vi "公式复合写入.vi"(11 "公式":cluster{"X^2":dbl, "X":dbl, "b":dbl}) -> ()   [LabVIEW 2016, in "斯坦道氨氮.lvlib"]
uses:
  <vilib>/Utility/miscctls.llb/LVPointTypeDef.ctl
panel:
  out "连接的字符串":string
  in  "参数下拉列表":enum16{"COD", "氨氮", "总氮", "总磷"}(ring)
  in  "量程下拉列表":enum16{"低量程", "高量程"}(ring)
  in  "取消":bool
  in  "确认":bool
  in  "加标回收":bool
  in  "标样核查":bool
  in  "跨度核查":bool
  in  "空白核查":bool
  in  "水样测量":bool=TRUE
  # "请选择要写入的参数"
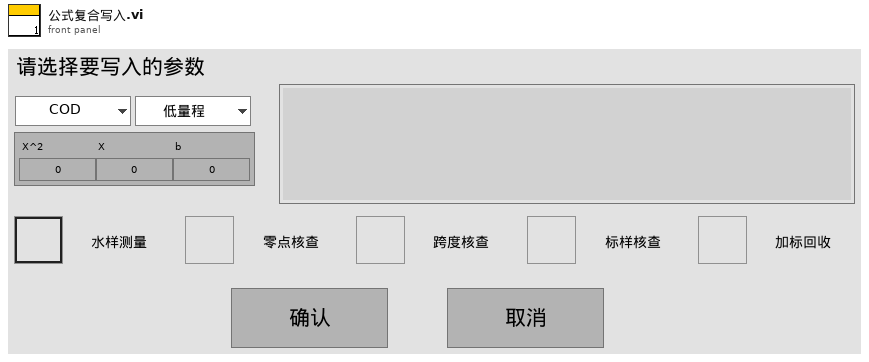
[diagram p1: front panel]
types:
  T1 = typedef "LVPointTypeDef.ctl" = cluster{"Horizontal":i16, "Vertical":i16}
  T2 = cluster{"COD":bool, "氨氮":bool, "总氮":bool, "总磷":bool}
  T3 = cluster{"测量量程":dbl, "测量精度":dbl, "测量间隔":dbl, "消解温度":dbl, "消解时长":dbl, "空白校准时间":timestamp, "曲线截距":dbl, "曲线斜率":dbl, "测量检出限":dbl, "测量信号值":dbl, "线性相关系数":dbl, "二次多项式系数":dbl, "标样校准时间":timestamp, "稀释倍数":dbl, "三项式系数":dbl, "空白标定系数":dbl, "量程系数":dbl, "F0/ORPA":dbl, "F1/ORPB":dbl, "F2/ORPK":dbl, "F3":dbl, "F4":dbl, "F5":dbl, "F6":dbl, "F7":dbl, "X0/滴定数":dbl, "量程":dbl}
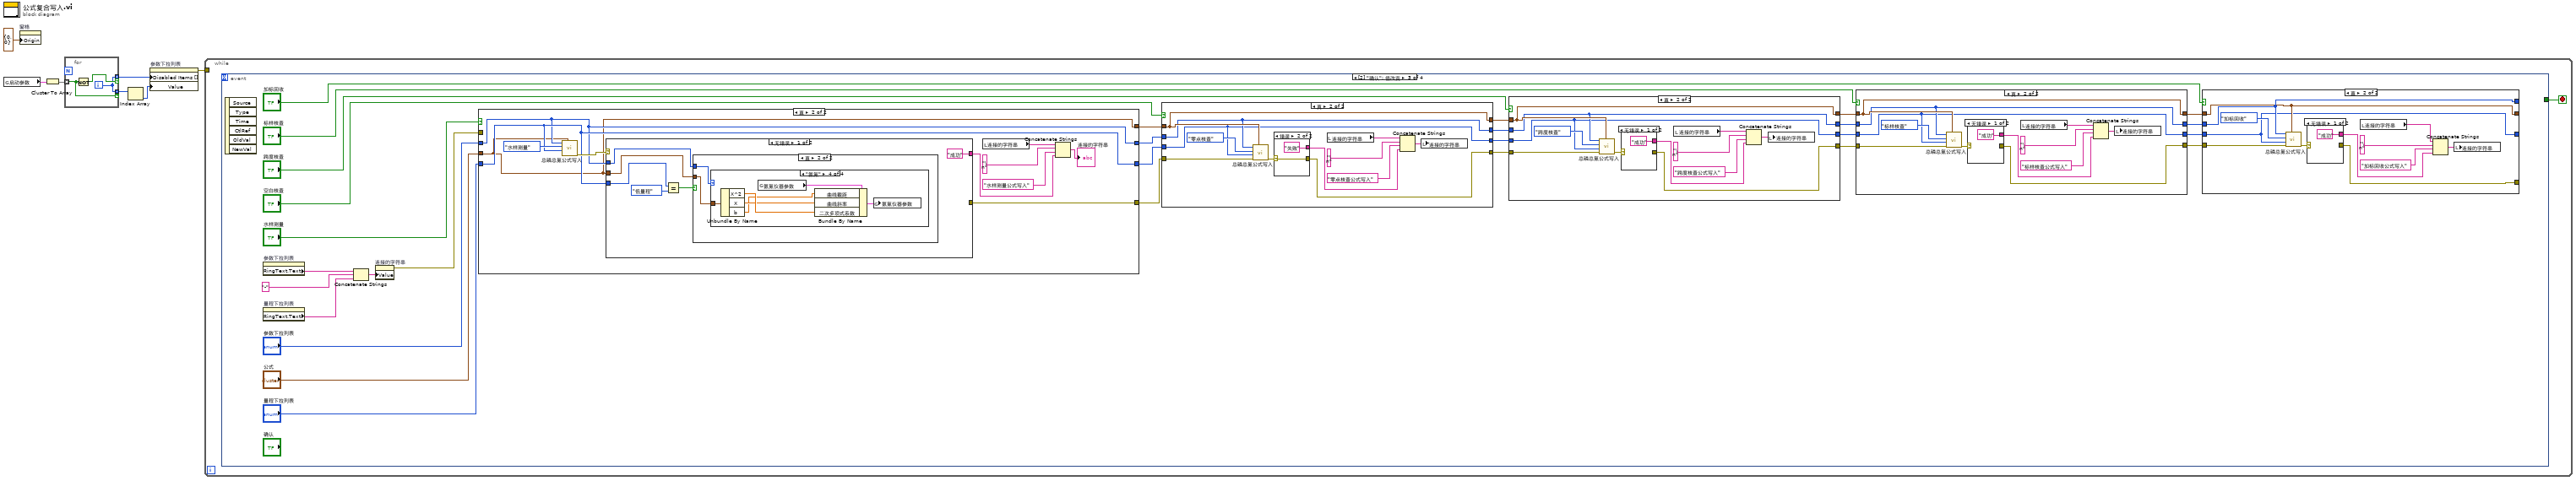
[diagram p0: block diagram]
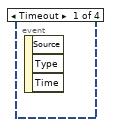
[diagram p2: hidden frame]
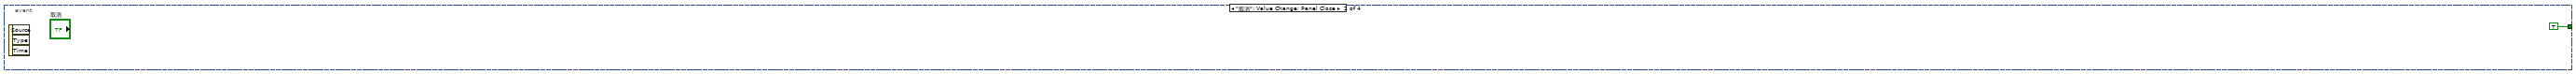
[diagram p3: hidden frame]
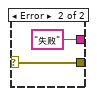
[diagram p5: hidden frame]
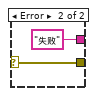
[diagram p7: hidden frame]
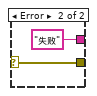
[diagram p9: hidden frame]
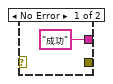
[diagram p11: hidden frame]
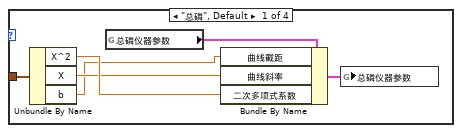
[diagram p14: hidden frame]
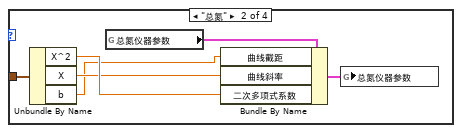
[diagram p15: hidden frame]
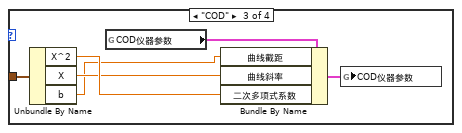
[diagram p16: hidden frame]
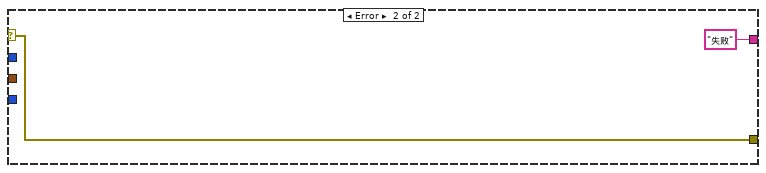
[diagram p17: hidden frame]
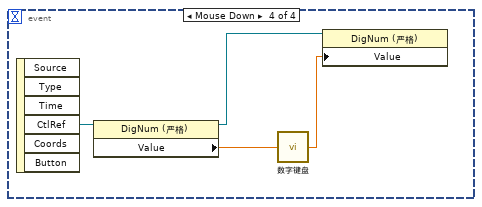
[diagram p18: hidden frame]
diagram:
  n1 = global read "总磷总氮断电保存全局变量.vi" "启动参数"() -> (w6:T2)
  n2 = property on="窗格" class="Pane"("Origin"=T1 {"Horizontal"=0, "Vertical"=0} ("原点")) -> ()  [unwired: 2 in, 2 out]
  n3 = Cluster To Array(cluster=w6) -> (array=w5:bool[])
  n4 = for {
    tunnel: w5 -> [w8] mode=indexing
    tunnel: [w9] -> w4 mode=indexing if=w10
    tunnel: [w9] -> w3 mode=indexing if=w8
    i -> [w9]
    n5 = Not(x=w8) -> (.not. x?=w10:bool)
  }
  n6 = Index Array(array=w3) -> (element=w2:i32)  [unwired: 1 in]
  n7 = property on="参数下拉列表" class="Enum (严格)"("Disabled Items []"=w4, "Value"=w2) -> (error out=w1:errorcluster)  [unwired: 2 in, 1 out]
  n8 = while {
    tunnel: w1 -> [_]
    stop <- w11 stop-if-true
    n9 = event shown="[2] \"确认\": 值改变" {
      selector: _ -> [_ _ _ _]
      dyn-events: _ -> [_ _ _ _]
      timeout: _ -> [_ _ _ _]
      tunnel: [_ TRUE _ _] -> w11
      event Timeout {
        n10 = event-data() -> ()  [unwired: 1 in, 3 out]
      }
      event "取消": Value Change; Panel Close {
        n11 = event-data() -> ()  [unwired: 1 in, 3 out]
      }
      event "确认": Value Change {
        n12 = event-data() -> ()  [unwired: 1 in, 6 out]
        n13 = property on="参数下拉列表" class="Enum (严格)"() -> ("RingText.Text"=w15:string)  [unwired: 2 in, 2 out]
        n14 = property on="量程下拉列表" class="Enum (严格)"() -> ("RingText.Text"=w14:string)  [unwired: 2 in, 2 out]
        n15 = Concatenate Strings(w15, "-" ("字符串"), w14) -> (w16:string)
        n16 = property on="连接的字符串" class="Str"("Value"=w16) -> (error out=w17:errorcluster)  [unwired: 2 in, 1 out]
        n17 = case shown="真" "水样测量" {
          tunnel: "公式" -> [w116 w117]
          tunnel: "参数下拉列表" -> [w115 w118]
          tunnel: "量程下拉列表" -> [w114 w119]
          tunnel: [w116 w117] -> w37
          tunnel: [w115 w118] -> w36
          tunnel: [w114 w119] -> w35
          tunnel: [_ w125] -> w19
          tunnel: w17 -> [_ _]
          frame False {
          }
          frame True {
            n18 = call "总磷总氮公式写入.vi"("公式"=w117, "量程"=w119, "测量模式"=enum16{"水样测量", "零点核查", "跨度核查", "标样核查", "加标回收"}."水样测量", "测量参数"=w118) -> ("error out"=w126:errorcluster)  [unwired: 7 in]
            n19 = case shown="无错误" w126 {
              selector: w126 -> [_ w161]
              tunnel: [_ w161] -> w125
              tunnel: ["成功" "失败"] -> w124
              tunnel: w119 -> [w132 _]
              tunnel: w118 -> [w129 _]
              tunnel: w117 -> [w128 _]
              frame No Error {
                n20 = Equal?(x=w132, y=enum16{"低量程", "高量程"}."低量程") -> (x = y?=w130:bool)
                n21 = case shown="真" w130 {
                  tunnel: w129 -> [_ w135]
                  tunnel: w128 -> [_ w134]
                  frame False {
                  }
                  frame True {
                    n22 = case shown="\"氨氮\"" w135 {
                      tunnel: w134 -> [w136 w142 w148 w154]
                      frame "总磷", Default {
                        n23 = Unbundle By Name(w136) -> ("X^2"=w139:dbl, "X"=w138:dbl, "b"=w137:dbl)
                        n24 = global read "总磷总氮断电保存全局变量.vi" "总磷仪器参数"() -> (w140:T3)
                        n25 = Bundle By Name(cluster=w140, "曲线截距"=w137, "曲线斜率"=w138, "二次多项式系数"=w139) -> (w141:T3)
                        n26 = global write "总磷总氮断电保存全局变量.vi" "总磷仪器参数"(w141) -> ()
                      }
                      frame "总氮" {
                        n27 = Unbundle By Name(w142) -> ("X^2"=w145:dbl, "X"=w144:dbl, "b"=w143:dbl)
                        n28 = global read "总磷总氮断电保存全局变量.vi" "总氮仪器参数"() -> (w146:T3)
                        n29 = Bundle By Name(cluster=w146, "曲线截距"=w143, "曲线斜率"=w144, "二次多项式系数"=w145) -> (w147:T3)
                        n30 = global write "总磷总氮断电保存全局变量.vi" "总氮仪器参数"(w147) -> ()
                      }
                      frame "COD" {
                        n31 = Unbundle By Name(w148) -> ("X^2"=w151:dbl, "X"=w150:dbl, "b"=w149:dbl)
                        n32 = global read "总磷总氮断电保存全局变量.vi" "COD仪器参数"() -> (w152:T3)
                        n33 = Bundle By Name(cluster=w152, "曲线截距"=w149, "曲线斜率"=w150, "二次多项式系数"=w151) -> (w153:T3)
                        n34 = global write "总磷总氮断电保存全局变量.vi" "COD仪器参数"(w153) -> ()
                      }
                      frame "氨氮" {
                        n35 = Unbundle By Name(w154) -> ("X^2"=w157:dbl, "X"=w156:dbl, "b"=w155:dbl)
                        n36 = global read "总磷总氮断电保存全局变量.vi" "氨氮仪器参数"() -> (w158:T3)
                        n37 = Bundle By Name(cluster=w158, "曲线截距"=w155, "曲线斜率"=w156, "二次多项式系数"=w157) -> (w159:T3)
                        n38 = global write "总磷总氮断电保存全局变量.vi" "氨氮仪器参数"(w159) -> ()
                      }
                    }
                  }
                }
              }
              frame Error {
              }
            }
            n39 = local read "连接的字符串"() -> (w121:string)
            n40 = Concatenate Strings(w121, "\n" ("字符串"), "水样测量公式写入", w124) -> (→"连接的字符串":string)
          }
        }
        n41 = case shown="真" "空白核查" {
          tunnel: w37 -> [w98 w109]
          tunnel: w36 -> [w97 w108]
          tunnel: w35 -> [w96 w107]
          tunnel: [_ w102] -> w34
          tunnel: [w98 w109] -> w33
          tunnel: [w97 w108] -> w32
          tunnel: [w96 w107] -> w31
          tunnel: w19 -> [_ w106]
          frame False {
          }
          frame True {
            n42 = call "总磷总氮公式写入.vi"("公式"=w109, "error in (no error)"=w106, "量程"=w107, "测量模式"=enum16{"水样测量", "零点核查", "跨度核查", "标样核查", "加标回收"}."零点核查", "测量参数"=w108) -> ("error out"=w103:errorcluster)  [unwired: 6 in]
            n43 = case shown="错误" w103 {
              selector: w103 -> [_ w113]
              tunnel: [_ w113] -> w102
              tunnel: ["成功" "失败"] -> w104
              frame No Error {
              }
              frame Error {
              }
            }
            n44 = local read "连接的字符串"() -> (w101:string)
            n45 = Concatenate Strings(w101, "\n" ("字符串"), "零点核查公式写入", w104) -> (w99:string)
            n46 = local write "连接的字符串"(w99) -> ()
          }
        }
        n47 = case shown="真" "跨度核查" {
          tunnel: w33 -> [w80 w91]
          tunnel: w32 -> [w79 w90]
          tunnel: w31 -> [w78 w89]
          tunnel: [w80 w91] -> w30
          tunnel: [w79 w90] -> w28
          tunnel: [w78 w89] -> w27
          tunnel: w34 -> [_ w88]
          tunnel: [_ w81] -> w18
          frame False {
          }
          frame True {
            n48 = call "总磷总氮公式写入.vi"("公式"=w91, "error in (no error)"=w88, "量程"=w89, "测量模式"=enum16{"水样测量", "零点核查", "跨度核查", "标样核查", "加标回收"}."跨度核查", "测量参数"=w90) -> ("error out"=w82:errorcluster)  [unwired: 6 in]
            n49 = case shown="无错误" w82 {
              selector: w82 -> [_ w95]
              tunnel: [_ w95] -> w81
              tunnel: ["成功" "失败"] -> w83
              frame No Error {
              }
              frame Error {
              }
            }
            n50 = local read "连接的字符串"() -> (w85:string)
            n51 = Concatenate Strings(w85, "\n" ("字符串"), "跨度核查公式写入", w83) -> (w87:string)
            n52 = local write "连接的字符串"(w87) -> ()
          }
        }
        n53 = case shown="真" "标样核查" {
          tunnel: w30 -> [w62 w73]
          tunnel: w28 -> [w61 w72]
          tunnel: w27 -> [w60 w71]
          tunnel: [_ w63] -> w24
          tunnel: [w62 w73] -> w29
          tunnel: [w61 w72] -> w26
          tunnel: [w60 w71] -> w25
          tunnel: w18 -> [_ w70]
          frame False {
          }
          frame True {
            n54 = call "总磷总氮公式写入.vi"("公式"=w73, "error in (no error)"=w70, "量程"=w71, "测量模式"=enum16{"水样测量", "零点核查", "跨度核查", "标样核查", "加标回收"}."标样核查", "测量参数"=w72) -> ("error out"=w64:errorcluster)  [unwired: 6 in]
            n55 = case shown="无错误" w64 {
              selector: w64 -> [_ w77]
              tunnel: [_ w77] -> w63
              tunnel: ["成功" "失败"] -> w65
              frame No Error {
              }
              frame Error {
              }
            }
            n56 = local read "连接的字符串"() -> (w67:string)
            n57 = Concatenate Strings(w67, "\n" ("字符串"), "标样核查公式写入", w65) -> (w69:string)
            n58 = local write "连接的字符串"(w69) -> ()
          }
        }
        n59 = case shown="真" "加标回收" {
          tunnel: w29 -> [w44 w55]
          tunnel: w26 -> [w43 w54]
          tunnel: w25 -> [w42 w53]
          tunnel: [w44 w55] -> _
          tunnel: [w43 w54] -> _
          tunnel: [w42 w53] -> _
          tunnel: w24 -> [_ w52]
          tunnel: [_ w45] -> _
          frame False {
          }
          frame True {
            n60 = call "总磷总氮公式写入.vi"("公式"=w55, "error in (no error)"=w52, "量程"=w53, "测量模式"=enum16{"水样测量", "零点核查", "跨度核查", "标样核查", "加标回收"}."加标回收", "测量参数"=w54) -> ("error out"=w46:errorcluster)  [unwired: 6 in]
            n61 = case shown="无错误" w46 {
              selector: w46 -> [_ w59]
              tunnel: [_ w59] -> w45
              tunnel: ["成功" "失败"] -> w47
              frame No Error {
              }
              frame Error {
              }
            }
            n62 = local read "连接的字符串"() -> (w49:string)
            n63 = Concatenate Strings(w49, "\n" ("字符串"), "加标回收公式写入", w47) -> (w51:string)
            n64 = local write "连接的字符串"(w51) -> ()
          }
        }
      }
      event "公式.X^2", "公式.X", "公式.b": Mouse Down {
        n65 = event-data() -> ("CtlRef"=w165:refnum<vi>)  [unwired: 1 in, 5 out]
        n66 = property class="DigNum (严格)"(reference=w165) -> (reference out=w162:refnum<vi>, "Value"=w164:dbl)  [unwired: 1 in, 1 out]
        n67 = call "数字键盘.vi"("OldNumber"=w164) -> ("NewNumber"=w163:dbl)
        n68 = property class="DigNum (严格)"(reference=w162, "Value"=w163) -> ()  [unwired: 1 in, 2 out]
      }
    }
  }
